vi "CheckMCP.vi"(2 "MCP Control Name":string, 3 "MCP_DIM_SetData":refnum<vi>[](array[refnum])) -> (0 "No Link?":bool, 1 "Safe?":bool)   [LabVIEW 2014, in "Panels.lvlib"]
uses:
  Panels.lvlib
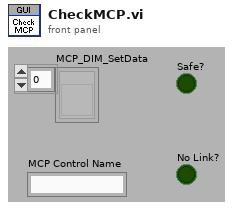
[diagram p1: front panel]
types:
  T1 = cluster{"data":dbl[], "no link":bool, "quality":i32, "timeStamp":dbl}
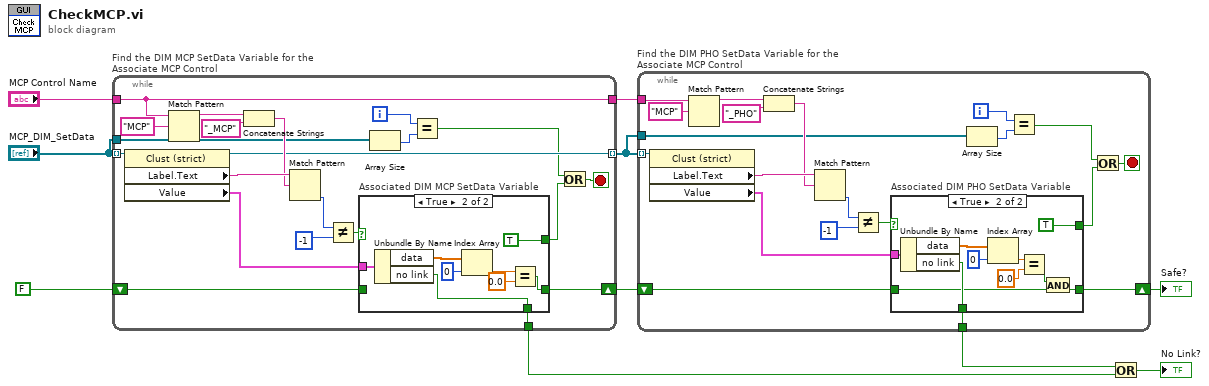
[diagram p0: block diagram]
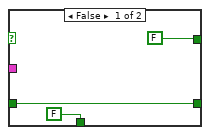
[diagram p2: hidden frame]
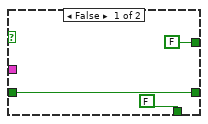
[diagram p3: hidden frame]
diagram:
  n1 = while "Find the DIM MCP SetData Variable for the Associate MCP Control" {
    tunnel: "MCP_DIM_SetData" -> [w26] mode=indexing
    tunnel: "MCP Control Name" -> [w19]
    shift-right: [w17] -> w6
    shift-left: FALSE ("no link") -> [w24]
    tunnel: [w20] -> w4 mode=indexing
    tunnel: [w19] -> w5
    tunnel: [w18] -> w1
    tunnel: "MCP_DIM_SetData" -> [w14]
    i -> [w12]
    stop <- w16 stop-if-true
    n2 = property class="Clust (strict)"(reference=w26) -> (reference out=w20:refnum<vi>, "Label.Text"=w30:string, "Value"=w27:T1)  [unwired: 1 in, 1 out]
    n3 = Match Pattern(string=w19, regular expression="MCP") -> (before substring=w23:string)  [unwired: 1 in, 3 out]
    n4 = Concatenate Strings(w23, "_MCP" ("string")) -> (w21:string)
    n5 = Match Pattern(string=w30, regular expression=w21) -> (offset past match=w29:i32)  [unwired: 1 in, 3 out]
    n6 = Not Equal?(x=w29, y=-1) -> (x != y?=w25:bool)
    n7 = case "Associated DIM MCP SetData Variable" shown="True" w25 {
      tunnel: w27 -> [_ w42]
      tunnel: w24 -> [w32 _]
      tunnel: [FALSE w37] -> w18
      tunnel: [FALSE TRUE] -> w15
      tunnel: [w32 w35] -> w17
      frame False {
      }
      frame True {
        n8 = Unbundle By Name(w42) -> ("data"=w41:dbl[], "no link"=w37:bool)
        n9 = Index Array(array=w41, index=0) -> (element=w40:dbl)
        n10 = Equal?(x=w40, y=0.0) -> (x = y?=w35:bool)
      }
    }
    n11 = Array Size(array=w14) -> (size(s)=w13:i32)
    n12 = Equal?(x=w12, y=w13) -> (x = y?=w11:bool)
    n13 = Or(x=w11, y=w15) -> (x .or. y?=w16:bool)
  }
  n14 = while "Find the DIM PHO SetData Variable for the Associate MCP Control" {
    tunnel: w4 -> [w57] mode=indexing
    shift-right: [w55] -> w7
    shift-left: w6 -> [w43]
    tunnel: w5 -> [w51]
    tunnel: [w50] -> w2
    tunnel: w4 -> [w48]
    i -> [w47]
    stop <- w46 stop-if-true
    n15 = property class="Clust (strict)"(reference=w57) -> ("Label.Text"=w61:string, "Value"=w58:T1)  [unwired: 1 in, 2 out]
    n16 = Match Pattern(string=w51, regular expression="MCP") -> (before substring=w54:string)  [unwired: 1 in, 3 out]
    n17 = Concatenate Strings(w54, "_PHO" ("string")) -> (w52:string)
    n18 = Match Pattern(string=w61, regular expression=w52) -> (offset past match=w60:i32)  [unwired: 1 in, 3 out]
    n19 = Not Equal?(x=w60, y=-1) -> (x != y?=w56:bool)
    n20 = case "Associated DIM PHO SetData Variable" shown="True" w56 {
      tunnel: w58 -> [_ w75]
      tunnel: [w63 w68] -> w55
      tunnel: [FALSE ("no link") w70] -> w50
      tunnel: [FALSE TRUE] -> w45
      tunnel: w43 -> [w63 w66]
      frame False {
      }
      frame True {
        n21 = Unbundle By Name(w75) -> ("data"=w74:dbl[], "no link"=w70:bool)
        n22 = Index Array(array=w74, index=0) -> (element=w73:dbl)
        n23 = Equal?(x=w73, y=0.0) -> (x = y?=w67:bool)
        n24 = And(x=w67, y=w66) -> (x .and. y?=w68:bool)
      }
    }
    n25 = Array Size(array=w48) -> (size(s)=w49:i32)
    n26 = Equal?(x=w47, y=w49) -> (x = y?=w44:bool)
    n27 = Or(x=w44, y=w45) -> (x .or. y?=w46:bool)
  }
  "Safe?" <- w7
  n28 = Or(x=w2, y=w1) -> (x .or. y?=→"No Link?":bool)
